vi "通道配置模块.vi"() -> ()   [LabVIEW 2010]
uses:
  <vilib>/Utility/config.llb/Write Key (String).vi
  <vilib>/Utility/config.llb/NI_LVConfig.lvlib
panel:
  out "配置文件路径":path
  out "配置文件目录":path
  in  "btn_保存配置":bool
  in  "加载配置文件列表":u16(ring) items=["5.ini", "5555.ini", "5896633sssss.ini", "7898.ini", "7898sssssss.ini", "789ddd8.ini"]
  in  "保存配置文件名称":string
  in  "btn_返回":bool
  in  "选项卡控件":T1(tab)
  in  "D_IN_1":string[][](table) caption="表格"
  in  "D_IN_2":string[][](table) caption="表格"
  in  "D_IN_3":string[][](table) caption="表格"
  in  "D_IN_4":string[][](table) caption="表格"
  # "控制板通道及参数配置"
  # "保存配置文件名称："
  # "加载配置文件："
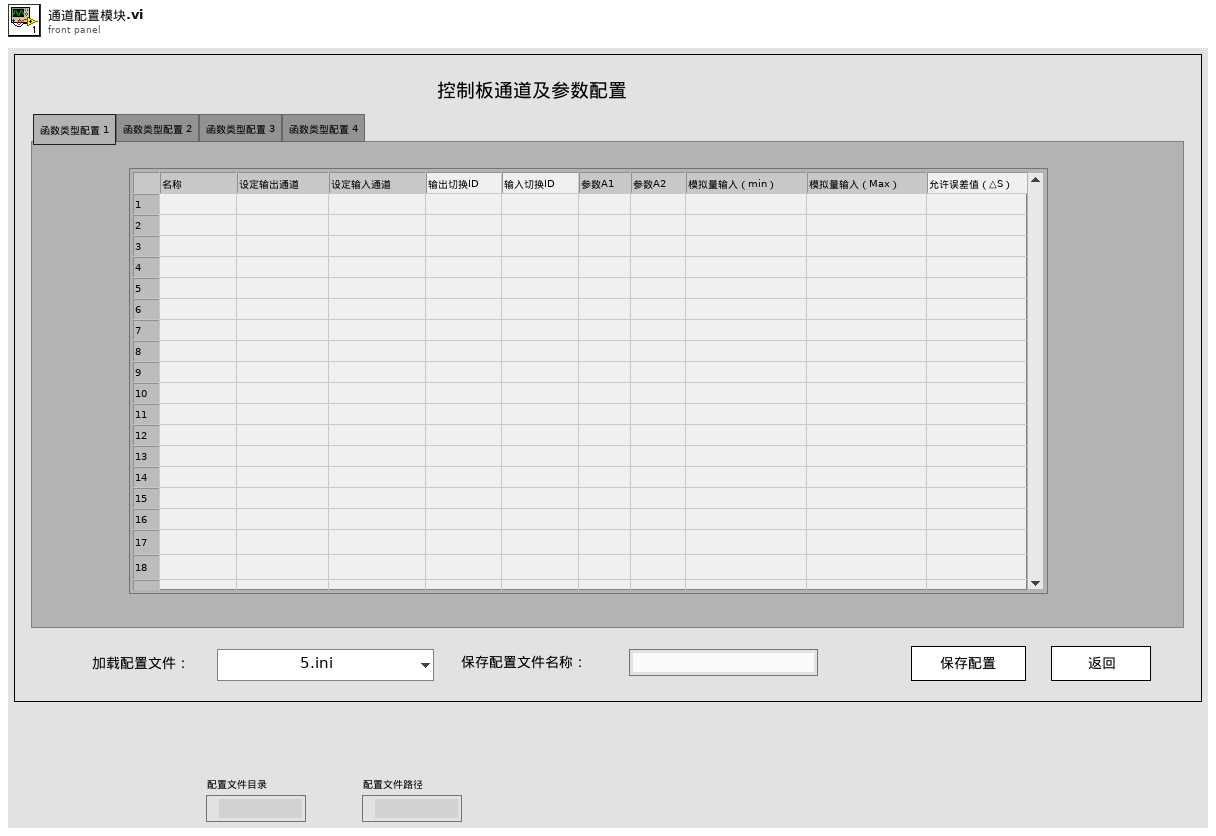
[diagram p1: front panel]
types:
  T1 = enum32{"函数类型配置 1", "函数类型配置 2", "函数类型配置 3", "函数类型配置 4"}
  T2 = typedef "NI_LVConfig.lvlib/Config Data RefNum.ctl" = refnum<k1>
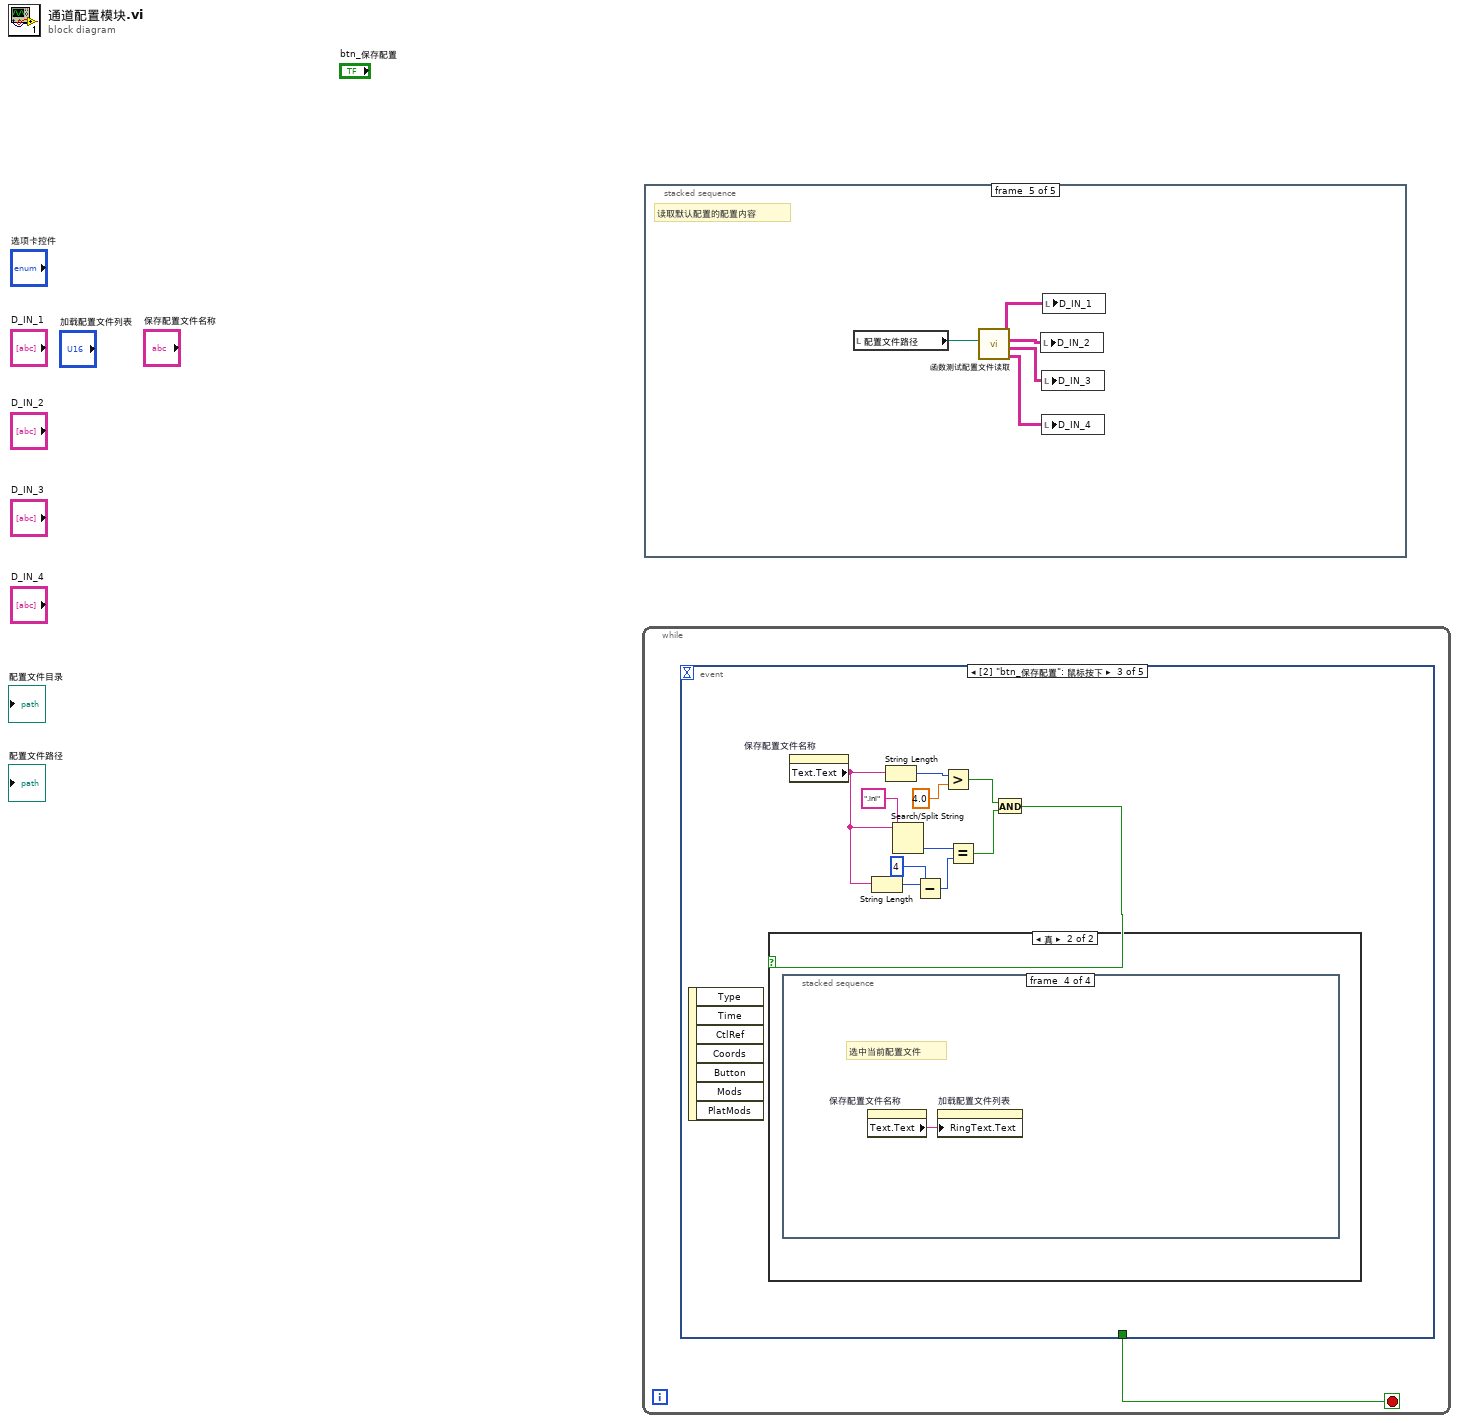
[diagram p0: block diagram]
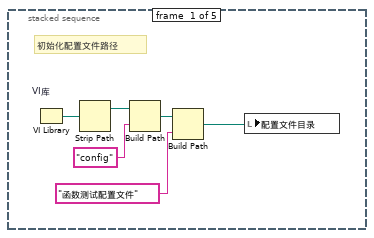
[diagram p2: hidden frame]
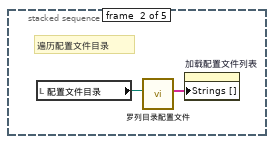
[diagram p3: hidden frame]
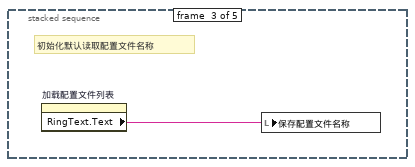
[diagram p4: hidden frame]
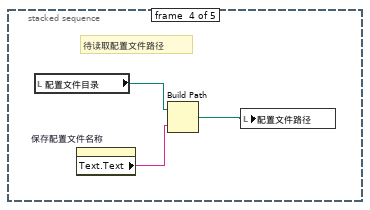
[diagram p5: hidden frame]
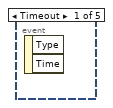
[diagram p6: hidden frame]
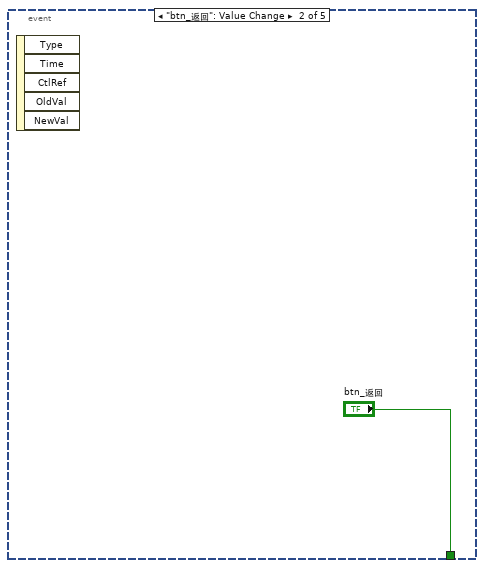
[diagram p7: hidden frame]
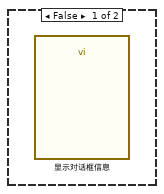
[diagram p8: hidden frame]
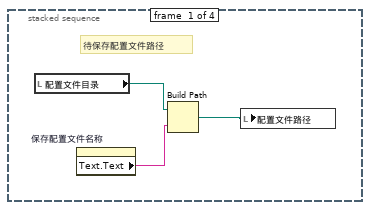
[diagram p9: hidden frame]
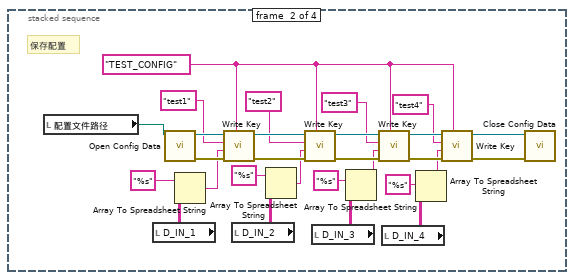
[diagram p10: hidden frame]
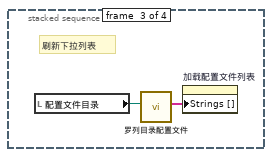
[diagram p11: hidden frame]
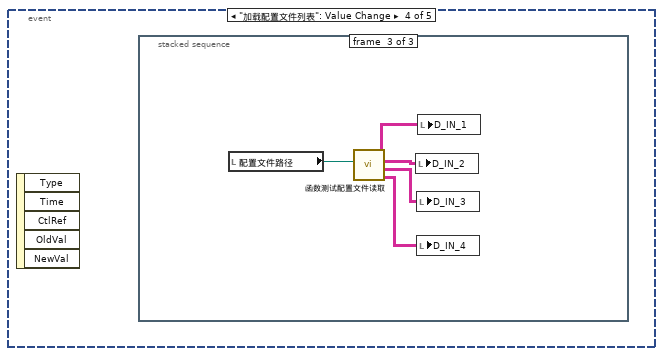
[diagram p12: hidden frame]
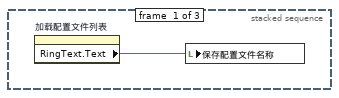
[diagram p13: hidden frame]
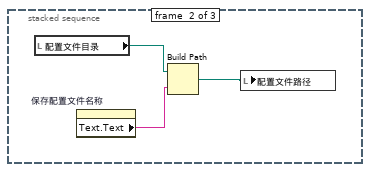
[diagram p14: hidden frame]
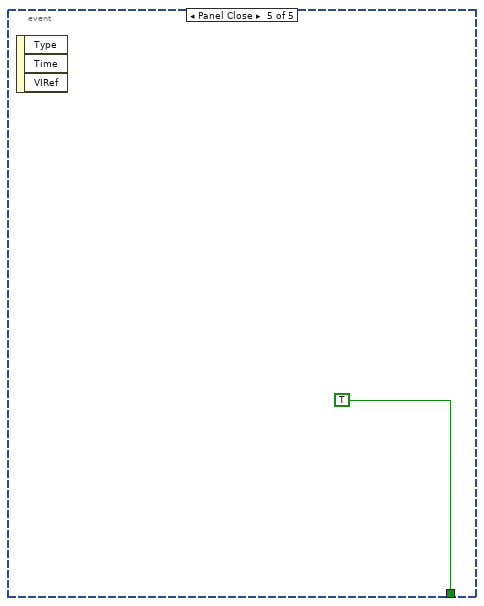
[diagram p15: hidden frame]
diagram:
  n1 = while {
    stop <- w1 stop-if-true
    n2 = event shown="[2] \"btn_保存配置\": 鼠标按下" {
      selector: _ -> [_ _ _ _ _]
      dyn-events: _ -> [_ _ _ _ _]
      timeout: _ -> [_ _ _ _ _]
      tunnel: [_ "btn_返回" _ _ TRUE] -> w1
      event Timeout {
        n3 = event-data() -> ()  [unwired: 1 in, 2 out]
      }
      event "btn_返回": Value Change {
        n4 = event-data() -> ()  [unwired: 1 in, 5 out]
      }
      event "btn_保存配置": Mouse Down {
        n5 = event-data() -> ()  [unwired: 1 in, 7 out]
        n6 = property on="保存配置文件名称" class="Str"() -> ("Text.Text"=w7:string)  [unwired: 2 in, 2 out]
        n7 = String Length(string=w7) -> (length=w6:i32)
        n8 = String Length(string=w7) -> (length=w11:i32)
        n9 = Search/Split String(string=w7, search string/char (-)=".ini" ("搜索字符串/字符(-)")) -> (offset of match=w8:i32)  [unwired: 1 in, 2 out]
        n10 = Subtract(x=w6, y=4) -> (x-y=w4:i32)
        n11 = Greater?(x=w11, y=4.0) -> (0:w10:bool)
        n12 = Equal?(x=w8, y=w4) -> (x = y?=w3:bool)
        n13 = And(x=w10, y=w3) -> (x .and. y?=w9:bool)
        n14 = case shown="真" w9 {
          frame False {
            n15 = call "显示对话框信息"() -> ()  [unwired: 10 in, 2 out]
          }
          frame True {
            n16 = stacked-sequence {
              frame #0 {
                # "待保存配置文件路径"
                n17 = local read "配置文件目录"() -> (w16:path)
                n18 = property on="保存配置文件名称" class="Str"() -> ("Text.Text"=w15:string)  [unwired: 2 in, 2 out]
                n19 = Build Path(base path=w16, name or relative path=w15) -> (appended path=w14:path)
                n20 = local write "配置文件路径"(w14) -> ()
              }
              frame #1 {
                w33 = "TEST_CONFIG" ("key")
                # "保存配置"
                n21 = local read "配置文件路径"() -> (w44:path)
                n22 = local read "D_IN_1"() -> (w35:string[][])
                n23 = call <vilib>:"Open Config Data.vi"("configuration file path"=w44) -> ("error out"=w43:errorcluster, "refnum"=w42:T2)  [unwired: 8 in, 1 out]
                n24 = Array To Spreadsheet String(array=w35, 3:"%s" ("格式字符串")) -> (spreadsheet string=w38:string)  [unwired: 1 in]
                n25 = call-poly <vilib>:"Write Key.vi"("section"=w33, "error in (no error)"=w43, "value"=w38, "key"="test1", "refnum"=w42) -> ("error out"=w41:errorcluster, "refnum out"=w40:T2)  [unwired: 4 in, 1 out]
                n26 = local read "D_IN_2"() -> (w36:string[][])
                n27 = Array To Spreadsheet String(array=w36, 3:"%s" ("格式字符串")) -> (spreadsheet string=w34:string)  [unwired: 1 in]
                n28 = call-poly <vilib>:"Write Key.vi"("section"=w33, "error in (no error)"=w41, "value"=w34, "key"="test2", "refnum"=w40) -> ("error out"=w29:errorcluster, "refnum out"=w32:T2)  [unwired: 4 in, 1 out]
                n29 = local read "D_IN_3"() -> (w24:string[][])
                n30 = Array To Spreadsheet String(array=w24, 3:"%s" ("格式字符串")) -> (spreadsheet string=w22:string)  [unwired: 1 in]
                n31 = call-poly <vilib>:"Write Key.vi"("section"=w33, "error in (no error)"=w29, "value"=w22, "key"="test3", "refnum"=w32) -> ("error out"=w28:errorcluster, "refnum out"=w31:T2)  [unwired: 4 in, 1 out]
                n32 = local read "D_IN_4"() -> (w23:string[][])
                n33 = Array To Spreadsheet String(array=w23, 3:"%s" ("格式字符串")) -> (spreadsheet string=w21:string)  [unwired: 1 in]
                n34 = call-poly <vilib>:"Write Key.vi"("section"=w33, "error in (no error)"=w28, "value"=w21, "key"="test4", "refnum"=w31) -> ("error out"=w27:errorcluster, "refnum out"=w30:T2)  [unwired: 4 in, 1 out]
                n35 = call <vilib>:"Close Config Data.vi"("error in (no error)"=w27, "refnum"=w30) -> ()  [unwired: 8 in, 2 out]
              }
              frame #2 {
                # "刷新下拉列表"
                n36 = local read "配置文件目录"() -> (w46:path)
                n37 = call "罗列目录配置文件.vi"("路径"=w46) -> ("数组"=w45:string[])  [unwired: 10 in]
                n38 = property on="加载配置文件列表" class="Ring (严格)"("Strings []"=w45) -> ()  [unwired: 2 in, 2 out]
              }
              frame #3 {
                # "选中当前配置文件"
                n39 = property on="保存配置文件名称" class="Str"() -> ("Text.Text"=w47:string)  [unwired: 2 in, 2 out]
                n40 = property on="加载配置文件列表" class="Ring (严格)"("RingText.Text"=w47) -> ()  [unwired: 2 in, 2 out]
              }
            }
          }
        }
      }
      event "加载配置文件列表": Value Change {
        n41 = event-data() -> ()  [unwired: 1 in, 5 out]
        n42 = stacked-sequence {
          frame #0 {
            n43 = property on="加载配置文件列表" class="Ring (严格)"() -> ("RingText.Text"=w48:string)  [unwired: 2 in, 2 out]
            n44 = local write "保存配置文件名称"(w48) -> ()
          }
          frame #1 {
            n45 = local read "配置文件目录"() -> (w51:path)
            n46 = property on="保存配置文件名称" class="Str"() -> ("Text.Text"=w50:string)  [unwired: 2 in, 2 out]
            n47 = Build Path(base path=w51, name or relative path=w50) -> (appended path=w49:path)
            n48 = local write "配置文件路径"(w49) -> ()
          }
          frame #2 {
            n49 = local read "配置文件路径"() -> (w52:path)
            n50 = call "函数测试配置文件读取.vi"("配置文件路径"=w52) -> ("D_IN_4"=w56:string[][], "D_IN_3"=w55:string[][], "D_IN_2"=w54:string[][], "D_IN_1"=w53:string[][])  [unwired: 6 in]
            n51 = local write "D_IN_2"(w54) -> ()
            n52 = local write "D_IN_3"(w55) -> ()
            n53 = local write "D_IN_4"(w56) -> ()
            n54 = local write "D_IN_1"(w53) -> ()
          }
        }
      }
      event Panel Close {
        n55 = event-data() -> ()  [unwired: 1 in, 3 out]
      }
    }
  }
  n56 = stacked-sequence {
    frame #0 {
      # "初始化配置文件路径"
      n57 = VI Library "VI库"() -> (path=w63:path)
      n58 = Strip Path(path=w63) -> (stripped path=w62:path)  [unwired: 1 out]
      n59 = Build Path(base path=w62, name or relative path="config" ("名称或相对路径")) -> (appended path=w60:path)
      n60 = Build Path(base path=w60, name or relative path="函数测试配置文件" ("名称或相对路径")) -> (appended path=w58:path)
      n61 = local write "配置文件目录"(w58) -> ()
    }
    frame #1 {
      # "遍历配置文件目录"
      n62 = local read "配置文件目录"() -> (w64:path)
      n63 = call "罗列目录配置文件.vi"("路径"=w64) -> ("数组"=w65:string[])  [unwired: 10 in]
      n64 = property on="加载配置文件列表" class="Ring (严格)"("Strings []"=w65) -> ()  [unwired: 2 in, 2 out]
    }
    frame #2 {
      # "初始化默认读取配置文件名称"
      n65 = property on="加载配置文件列表" class="Ring (严格)"() -> ("RingText.Text"=w66:string)  [unwired: 2 in, 2 out]
      n66 = local write "保存配置文件名称"(w66) -> ()
    }
    frame #3 {
      # "待读取配置文件路径"
      n67 = local read "配置文件目录"() -> (w67:path)
      n68 = property on="保存配置文件名称" class="Str"() -> ("Text.Text"=w68:string)  [unwired: 2 in, 2 out]
      n69 = Build Path(base path=w67, name or relative path=w68) -> (appended path=w69:path)
      n70 = local write "配置文件路径"(w69) -> ()
    }
    frame #4 {
      # "读取默认配置的配置内容"
      n71 = local read "配置文件路径"() -> (w74:path)
      n72 = call "函数测试配置文件读取.vi"("配置文件路径"=w74) -> ("D_IN_4"=w70:string[][], "D_IN_3"=w71:string[][], "D_IN_2"=w72:string[][], "D_IN_1"=w73:string[][])  [unwired: 6 in]
      n73 = local write "D_IN_2"(w72) -> ()
      n74 = local write "D_IN_3"(w71) -> ()
      n75 = local write "D_IN_4"(w70) -> ()
      n76 = local write "D_IN_1"(w73) -> ()
    }
  }
